vi "MotherBoard.vi"(8 "error in (no error)":errorcluster, 9 "Product_Ref":string) -> (0 "error out":errorcluster, 3 "Board out":refnum<class "Board.lvclass">)   [LabVIEW 2025, in "Board.lvclass"]
uses:
  Board.lvclass
  Board.lvclass/Board.ctl
  <vilib>/Utility/error.llb/Error Cluster From Error Code.vi
  <vilib>/ErrorRing/Error Ring.xnode
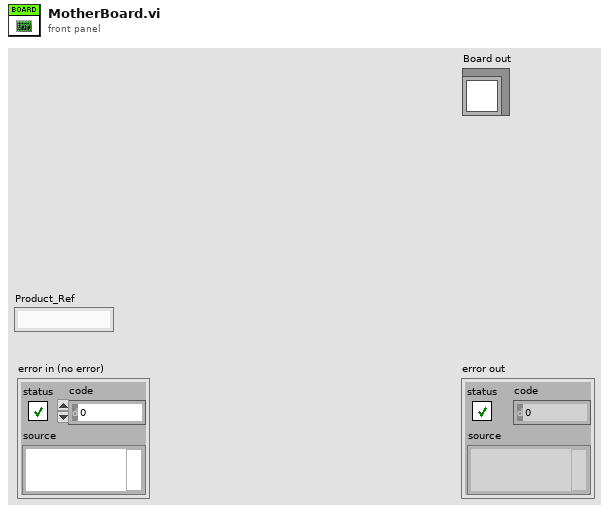
[diagram p1: front panel]
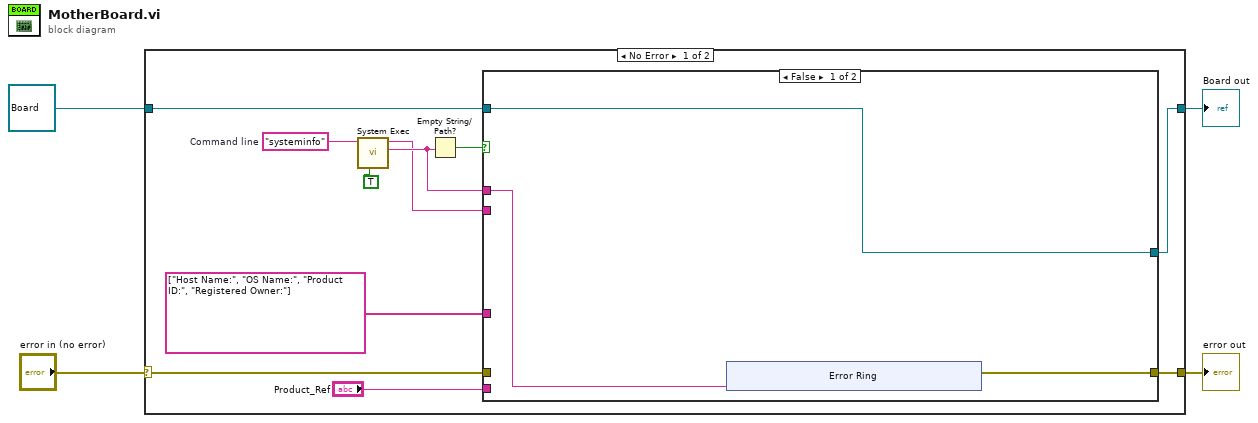
[diagram p0: block diagram]
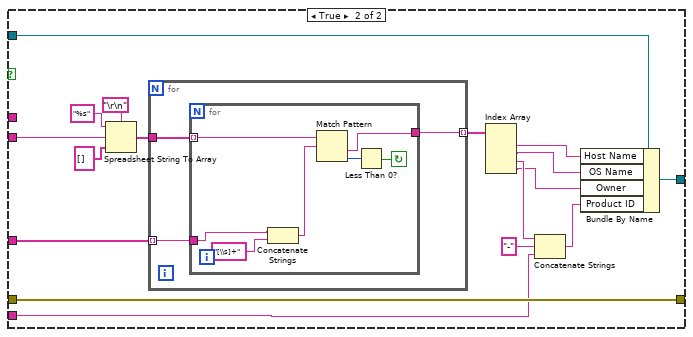
[diagram p2: hidden frame]
diagram:
  n1 = case shown="No Error" "error in (no error)" {
    selector: "error in (no error)" -> [w14 w54]
    tunnel: [w15 w54] -> w3
    tunnel: [w9 w53] -> w1
    tunnel: refnum<class "Board.lvclass"> refnum ("Board in") -> [w8 w53]
    frame No Error {
      w12 = "systeminfo"  # Command line
      n2 = call <vilib>:"System Exec.vi"("run minimized? (F)"=TRUE, "command line"=w12) -> ("standard error"=w11:string, "standard output"=w10:string)  [unwired: 6 in, 2 out]
      n3 = Empty String/Path?(string/path=w11) -> (empty?=w13:bool)
      n4 = case shown="False" w13 {
        tunnel: [w18 w42] -> w15
        tunnel: w14 -> [_ w42]
        tunnel: w11 -> [w17 _]
        tunnel: w10 -> [_ w35]
        tunnel: [w16 w40] -> w9
        tunnel: w8 -> [w16 w41]
        tunnel: string[] ["Host Name:", "OS Name:", "Product ID:", "Registered Owner:"] -> [_ w39]
        tunnel: "Product_Ref" -> [_ w26]
        frame False {
          n5 = xnode "Error Ring"("parameter 0"=w17) -> ("error out"=w18:errorcluster)
        }
        frame True {
          n6 = Spreadsheet String To Array(delimiter (Tab)="\r\n", format string="%s" ("String"), spreadsheet string=w35, array type (2D Dbl)=string[] []) -> (array=w37:string[])
          n7 = for {
            tunnel: w39 -> [w45] mode=indexing
            tunnel: w37 -> [w44]
            tunnel: [w43] -> w33 mode=indexing
            n8 = for {
              tunnel: w45 -> [w52]
              tunnel: w44 -> [w49] mode=indexing
              tunnel: [w46] -> w43
              stop <- w47 continue-if-true
              n9 = Concatenate Strings(w52, "[\\s]+" ("string")) -> (w50:string)
              n10 = Match Pattern(string=w49, regular expression=w50) -> (after substring=w46:string, offset past match=w48:i32)  [unwired: 1 in, 2 out]
              n11 = Less Than 0?(x=w48) -> (x < 0?=w47:bool)
            }
          }
          n12 = Index Array(array=w33) -> (element #1=w32:string, element #2=w31:string, element #3=w30:string, element #4=w29:string)  [unwired: 4 in]
          n13 = Concatenate Strings(w30, "-" ("string"), w26) -> (w28:string)
          n14 = Bundle By Name(cluster=w41, "Host Name"=w32, "OS Name"=w31, "Owner"=w29, "Product ID"=w28) -> (w40:refnum<class "Board.lvclass">)
        }
      }
    }
    frame Error {
    }
  }
  "error out" <- w3
  "Board out" <- w1
